vi "WPI_DriverStationGame Specific Data.vi"() -> (2 "Game Specific Data":string)   [LabVIEW 2017]
doc: "Returns game specific data from the FMS (Field Management System).\n\nThis software is licensed. Open the labview\\readme\\WPI Robotics Library Open Source License.txt file for more information."
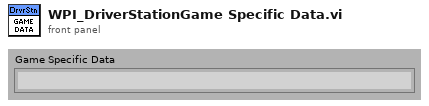
[diagram p1: front panel]
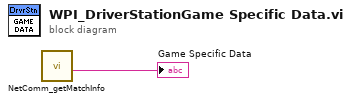
[diagram p0: block diagram]
diagram:
  n1 = call <vilib>:"NetComm_getMatchInfo.vi"() -> ("Game Specific Data"=→"Game Specific Data":string)  [unwired: 6 in, 5 out]
